vi "post math 2(SubVI).vi"(7 "tics in one rotation":dbl, 10 "WANTED (W)":dbl, 11 "refnum name":string="My Motor RefNum") -> (3 "positiony":dbl)   [LabVIEW 2020]
uses:
  <vilib>/Rock Robotics/WPI/ThirdParty/Phoenix-LabVIEW/Motor Controller/Get/CTRE_Phoenix_MotorController_GetSelectedSensorData.vi
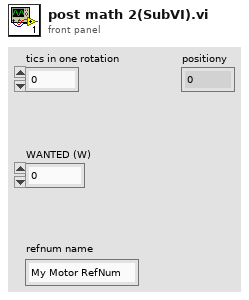
[diagram p1: front panel]
types:
  T1 = typedef "WPI_MotorControlDeviceRef.ctl" = cluster{"DeviceStatus":errorcluster, "Type":T2, "PWM":cluster{"PWM Channel":T3, "DeadBand":T4}, "CAN":cluster{"Device Number":u8, "SetOutput VI Ref":variant, "GetOutput VI Ref":variant, "Enable VI Ref":variant, "Disable VI Ref":variant, "Data":variant}, "Invert":bool, "DIO PWM":cluster{"PWM \"Enable\" Channel":T3, "DIOChannel":T5, "PWM Rate":dbl}}
  T2 = typedef "WPI_MotorControlType.ctl" = enum16{"PWM", "CAN", "DIO PWM"}
  T3 = typedef "FPGA_DIOPWMChannel.ctl" = enum8{"PWM 0", "PWM 1", "PWM 2", "PWM 3", "PWM 4", "PWM 5", "PWM 6", "PWM 7", "PWM 8", "PWM 9", "PWM MXP 0", "PWM MXP 1", "PWM MXP 2", "PWM MXP 3", "PWM MXP 4", "PWM MXP 5", "PWM MXP 6", "PWM MXP 7", "PWM MXP 8", "PWM MXP 9", "Invalid"}
  T4 = typedef "WPI_PWMDeadband.ctl" = cluster{"Name":string, "maxPositivePwm":i32, "minPositivePwm":i32, "centerPwm":i32, "maxNegativePwm":i32, "minNegativePwm":i32, "angularRange":u16}
  T5 = typedef "FPGA_DIOChannel.ctl" = enum8{"DIO 0", "DIO 1", "DIO 2", "DIO 3", "DIO 4", "DIO 5", "DIO 6", "DIO 7", "DIO 8", "DIO 9", "DIO MXP 0", "DIO MXP 1", "DIO MXP 2", "DIO MXP 3", "DIO MXP 4", "DIO MXP 5", "DIO MXP 6", "DIO MXP 7", "DIO MXP 8", "DIO MXP 9", "DIO MXP 10", "DIO MXP 11", "DIO MXP 12", "DIO MXP 13", "DIO MXP 14", "DIO MXP 15", "SPI Port CS1", "SPI Port CS2", "SPI Port CS3", "SPI Port MISO", "SPI Port MOSI", "Invalid"}
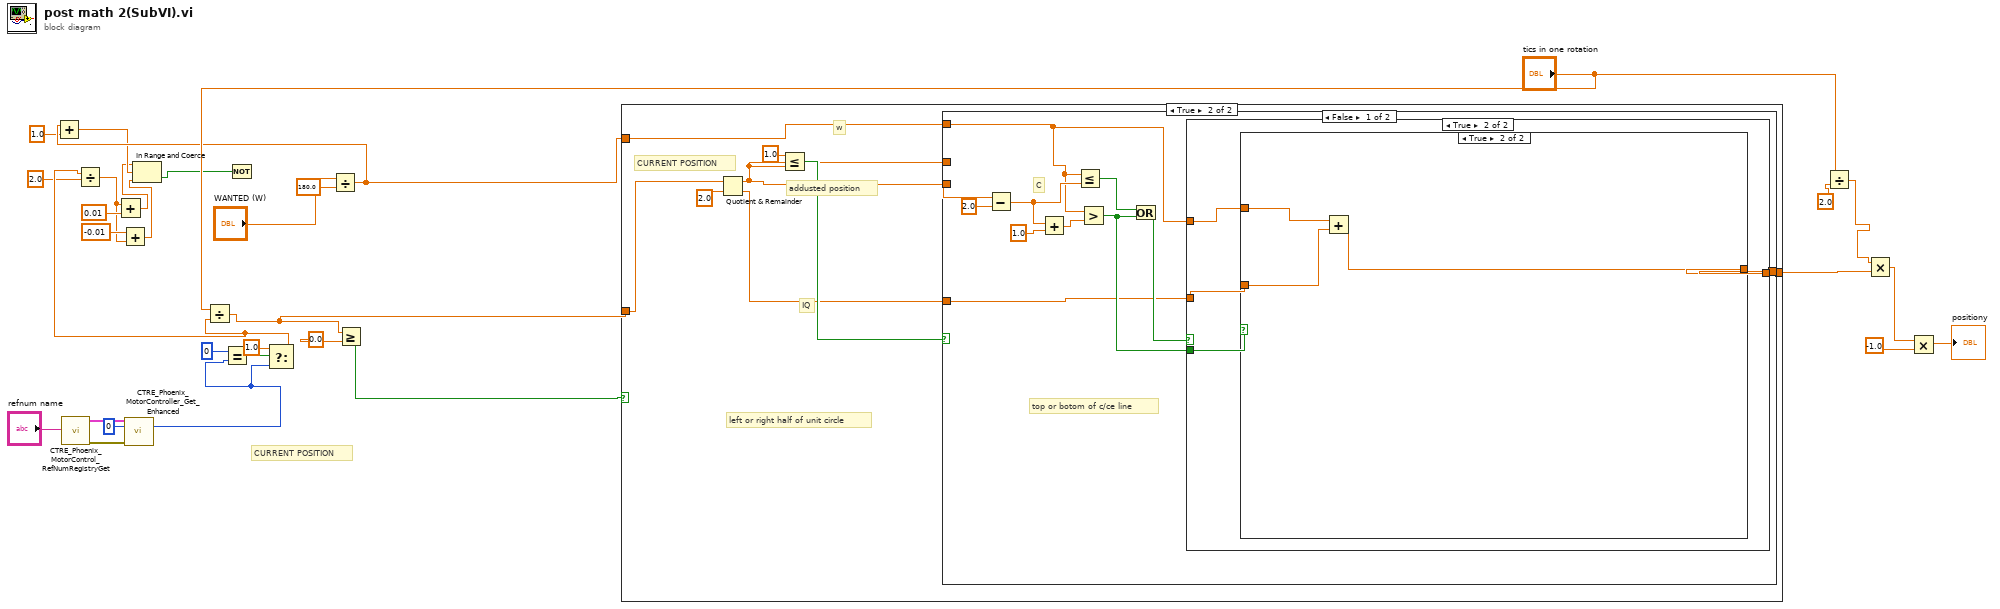
[diagram p0: block diagram]
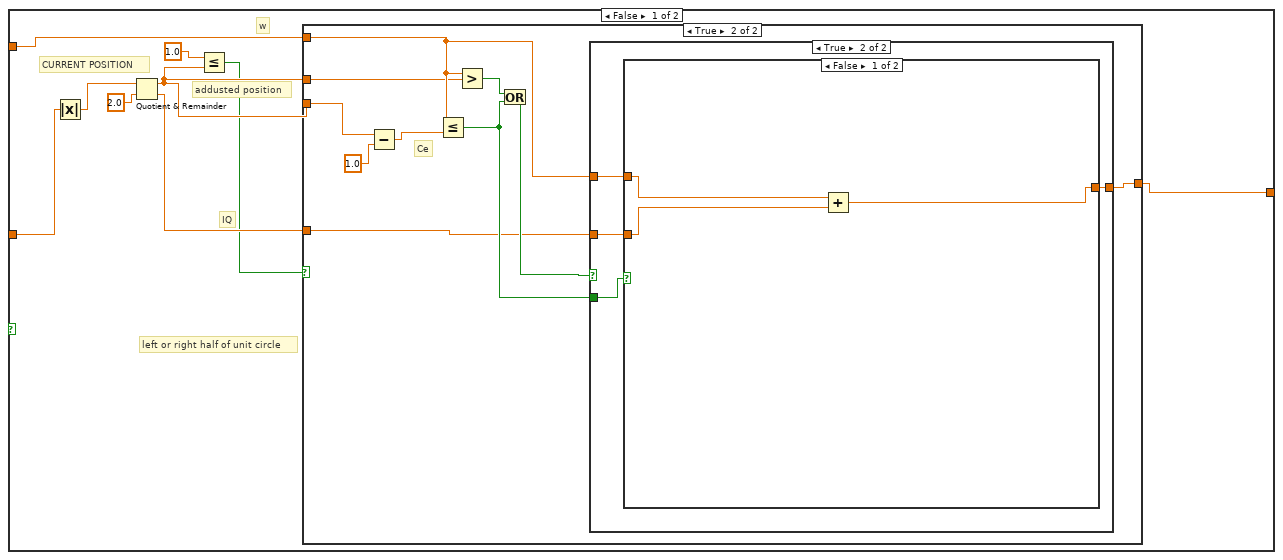
[diagram p2: hidden frame]
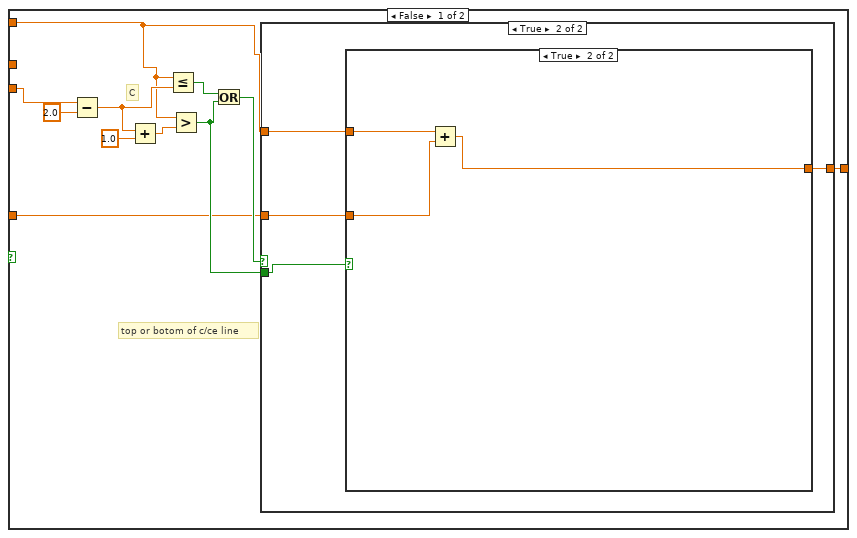
[diagram p3: hidden frame]
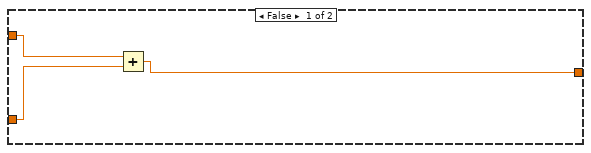
[diagram p4: hidden frame]
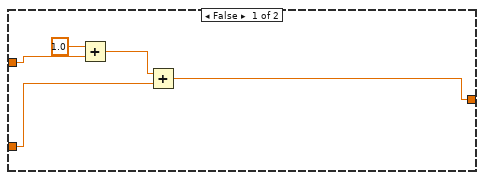
[diagram p5: hidden frame]
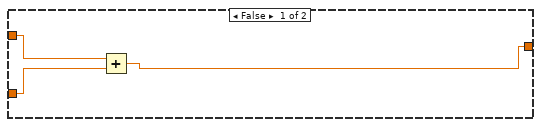
[diagram p6: hidden frame]
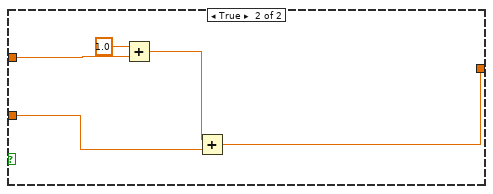
[diagram p7: hidden frame]
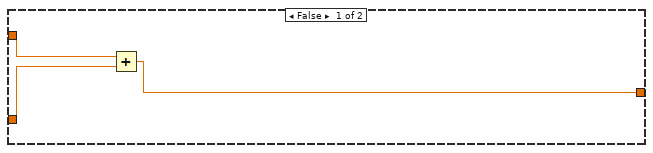
[diagram p8: hidden frame]
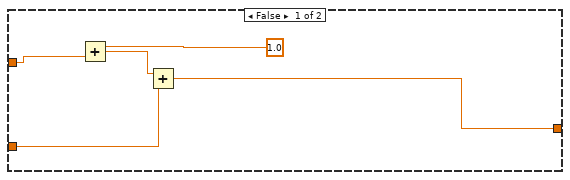
[diagram p9: hidden frame]
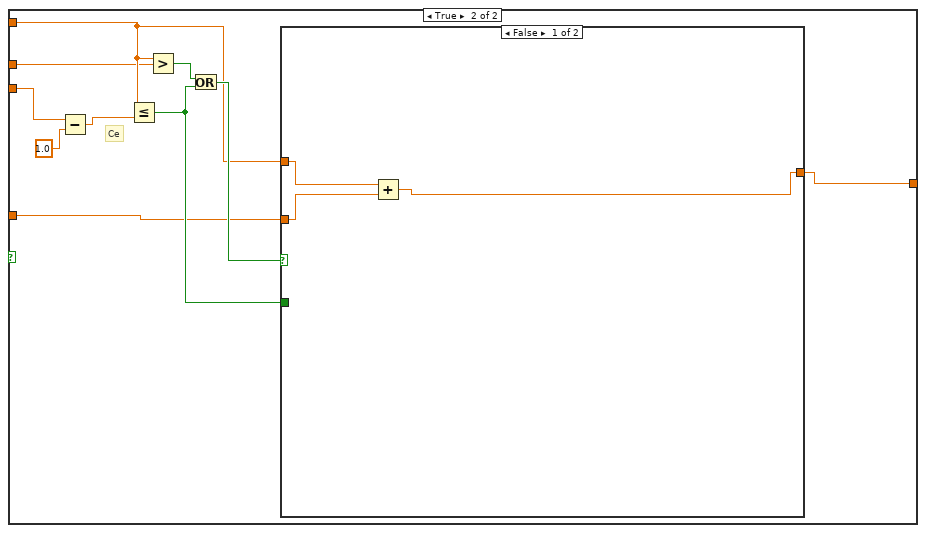
[diagram p10: hidden frame]
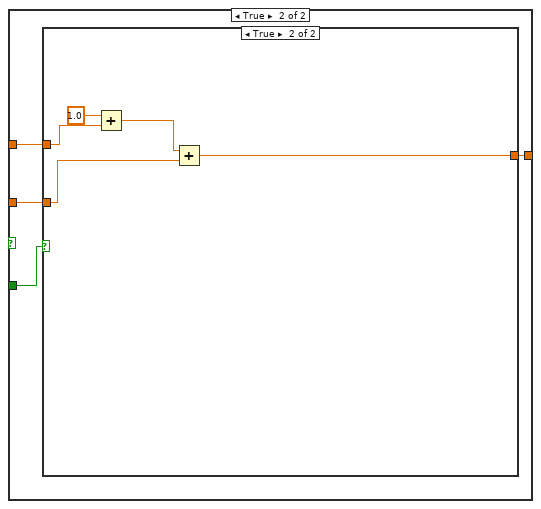
[diagram p11: hidden frame]
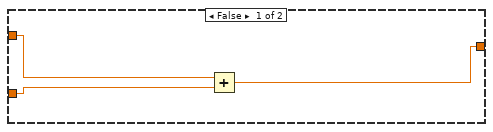
[diagram p12: hidden frame]
diagram:
  # "CURRENT POSITION"
  n1 = call <vilib>:"CTRE_Phoenix_MotorControl_RefNumRegistryGet.vi"("refnum name"="refnum name") -> ("error out"=w26:errorcluster, "PhoenixMotorControlDevRef"=w27:T1)  [unwired: 9 in]
  n2 = call-poly <vilib>:"CTRE_Phoenix_MotorController_Get_Enhanced.vi"("PhoenixMotorControlDevRef"=w27, "pidLoopIdx"=u32 0, "error in"=w26) -> ("Position (Raw Sensor Units)"=w14:i32)  [unwired: 9 in, 3 out]
  n3 = Equal?(x=0, y=w14) -> (x = y?=w16:bool)
  n4 = Select(t=1.0, s=w16, f=w14) -> (s? t:f=w11:dbl)
  n5 = Divide(x=w11, y=2.0) -> (x/y=w6:dbl)
  n6 = Add(x=w6, y=0.01) -> (x+y=w5:dbl)
  n7 = Add(x=-0.01, y=w6) -> (x+y=w4:dbl)
  n8 = Divide(x="tics in one rotation", y=w11) -> (x/y=w21:dbl)
  n9 = Divide(x="WANTED (W)", y=180.0) -> (x/y=w13:dbl)
  n10 = Add(x=w13, y=1.0) -> (x+y=w9:dbl)
  n11 = In Range and Coerce(upper limit=w5, x=w9, lower limit=w4) -> (In Range?=w3:bool)  [unwired: 1 out]
  n12 = Not(x=w3) -> ()  [unwired: 1 out]
  n13 = Greater Or Equal?(x=w21, y=0.0) -> (x >= y?=w24:bool)
  n14 = case shown="True" w24 {
    tunnel: w13 -> [w35 w96]
    tunnel: [w33 w94] -> w25
    tunnel: w21 -> [w32 w92]
    frame False {
      # "left or right half of unit circle"
      # "w"
      # "IQ"
      # "addusted position"
      # "CURRENT POSITION"
      n15 = Absolute Value(x=w32) -> (abs(x)=w34:dbl)
      n16 = Quotient & Remainder(x=w34, y=2.0) -> (x-y*floor(x/y)=w40:dbl, floor(x/y)=w39:dbl)
      n17 = Less Or Equal?(x=1.0, y=w40) -> (x <= y?=w38:bool)
      n18 = case shown="True" w38 {
        tunnel: w40 -> [_ w70]
        tunnel: w35 -> [w43 w73]
        tunnel: w39 -> [w42 w72]
        tunnel: [w41 w71] -> w33
        tunnel: w40 -> [w51 w69]
        frame False {
          # "top or botom of c/ce line"
          # "C"
          n19 = Subtract(x=w51, y=2.0) -> (x-y=w49:dbl)
          n20 = Add(x=w49, y=1.0) -> (x+y=w47:dbl)
          n21 = Less Or Equal?(x=w43, y=w49) -> (x <= y?=w46:bool)
          n22 = Greater?(x=w43, y=w47) -> (0:w44:bool)
          n23 = Or(x=w46, y=w44) -> (x .or. y?=w45:bool)
          n24 = case shown="True" w45 {
            tunnel: w44 -> [_ w58]
            tunnel: w43 -> [w54 w57]
            tunnel: w42 -> [w53 w56]
            tunnel: [w52 w55] -> w41
            frame False {
              n25 = Add(x=w54, y=w53) -> (x+y=w52:dbl)
            }
            frame True {
              n26 = case shown="True" w58 {
                tunnel: w57 -> [w63 w66]
                tunnel: w56 -> [w60 w65]
                tunnel: [w59 w64] -> w55
                frame False {
                  n27 = Add(x=1.0, y=w63) -> (x+y=w61:dbl)
                  n28 = Add(x=w61, y=w60) -> (x+y=w59:dbl)
                }
                frame True {
                  n29 = Add(x=w66, y=w65) -> (x+y=w64:dbl)
                }
              }
            }
          }
        }
        frame True {
          # "Ce"
          n30 = Subtract(x=w69, y=1.0) -> (x-y=w68:dbl)
          n31 = Less Or Equal?(x=w73, y=w68) -> (x <= y?=w74:bool)
          n32 = Greater?(x=w73, y=w70) -> (0:w76:bool)
          n33 = Or(x=w76, y=w74) -> (x .or. y?=w75:bool)
          n34 = case shown="True" w75 {
            tunnel: w74 -> [_ w83]
            tunnel: w73 -> [w79 w82]
            tunnel: w72 -> [w78 w81]
            tunnel: [w77 w80] -> w71
            frame False {
              n35 = Add(x=w79, y=w78) -> (x+y=w77:dbl)
            }
            frame True {
              n36 = case shown="False" w83 {
                tunnel: w82 -> [w85 w91]
                tunnel: w81 -> [w86 w88]
                tunnel: [w84 w87] -> w80
                frame False {
                  n37 = Add(x=w85, y=w86) -> (x+y=w84:dbl)
                }
                frame True {
                  n38 = Add(x=1.0, y=w91) -> (x+y=w89:dbl)
                  n39 = Add(x=w89, y=w88) -> (x+y=w87:dbl)
                }
              }
            }
          }
        }
      }
    }
    frame True {
      # "left or right half of unit circle"
      # "w"
      # "IQ"
      # "addusted position"
      # "CURRENT POSITION"
      n40 = Quotient & Remainder(x=w92, y=2.0) -> (x-y*floor(x/y)=w93:dbl, floor(x/y)=w95:dbl)
      n41 = Less Or Equal?(x=1.0, y=w93) -> (x <= y?=w97:bool)
      n42 = case shown="False" w97 {
        tunnel: w93 -> [_ w129]
        tunnel: w96 -> [w102 w132]
        tunnel: w95 -> [w101 w131]
        tunnel: [w100 w130] -> w94
        tunnel: w93 -> [w110 w128]
        frame False {
          # "top or botom of c/ce line"
          # "C"
          n43 = Subtract(x=w110, y=2.0) -> (x-y=w108:dbl)
          n44 = Add(x=w108, y=1.0) -> (x+y=w106:dbl)
          n45 = Less Or Equal?(x=w102, y=w108) -> (x <= y?=w105:bool)
          n46 = Greater?(x=w102, y=w106) -> (0:w103:bool)
          n47 = Or(x=w105, y=w103) -> (x .or. y?=w104:bool)
          n48 = case shown="True" w104 {
            tunnel: w103 -> [_ w117]
            tunnel: w102 -> [w113 w116]
            tunnel: w101 -> [w112 w115]
            tunnel: [w111 w114] -> w100
            frame False {
              n49 = Add(x=w113, y=w112) -> (x+y=w111:dbl)
            }
            frame True {
              n50 = case shown="True" w117 {
                tunnel: w116 -> [w122 w125]
                tunnel: w115 -> [w119 w124]
                tunnel: [w118 w123] -> w114
                frame False {
                  n51 = Add(x=1.0, y=w122) -> (x+y=w120:dbl)
                  n52 = Add(x=w120, y=w119) -> (x+y=w118:dbl)
                }
                frame True {
                  n53 = Add(x=w125, y=w124) -> (x+y=w123:dbl)
                }
              }
            }
          }
        }
        frame True {
          # "Ce"
          n54 = Subtract(x=w128, y=1.0) -> (x-y=w127:dbl)
          n55 = Less Or Equal?(x=w132, y=w127) -> (x <= y?=w133:bool)
          n56 = Greater?(x=w132, y=w129) -> (0:w135:bool)
          n57 = Or(x=w135, y=w133) -> (x .or. y?=w134:bool)
          n58 = case shown="False" w134 {
            tunnel: w133 -> [_ w142]
            tunnel: w132 -> [w138 w141]
            tunnel: w131 -> [w137 w140]
            tunnel: [w136 w139] -> w130
            frame False {
              n59 = Add(x=w138, y=w137) -> (x+y=w136:dbl)
            }
            frame True {
              n60 = case shown="True" w142 {
                tunnel: w141 -> [w145 w150]
                tunnel: w140 -> [w143 w147]
                tunnel: [w144 w146] -> w139
                frame False {
                  n61 = Add(x=w145, y=w143) -> (x+y=w144:dbl)
                }
                frame True {
                  n62 = Add(x=1.0, y=w150) -> (x+y=w148:dbl)
                  n63 = Add(x=w148, y=w147) -> (x+y=w146:dbl)
                }
              }
            }
          }
        }
      }
    }
  }
  n64 = Divide(x="tics in one rotation", y=2.0) -> (x/y=w20:dbl)
  n65 = Multiply(x=w20, y=w25) -> (x*y=w1:dbl)
  n66 = Multiply(x=w1, y=-1.0) -> (x*y=→"positiony":dbl)
